vi "Configure Numeric Preset.vi"(8 "error in (no error)":errorcluster, 9 "Preset (Pattern 1)":i32(ring)=1 items=["Pattern 1"=1, "Pattern 2"=2, "Pattern 3"=3, "Pattern 4"=4], 10 "Target Item (0: Normal)":i32(ring) items=["Normal", "Harmonics"], 11 "VISA resource name":refnum<visa-resource-name>) -> (0 "error out":errorcluster, 3 "VISA resource name out":refnum<visa-resource-name>)   [LabVIEW 2021, in "Yokogawa WT1800 Series.lvlib"]
doc: "Configures the numeric preset features."
uses:
  <instrlib>/Yokogawa WT1800 Series/Yokogawa WT1800 Series.lvlib
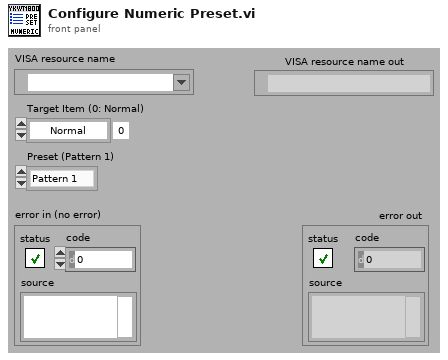
[diagram p1: front panel]
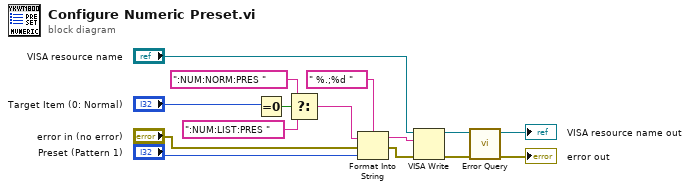
[diagram p0: block diagram]
diagram:
  n1 = Equal To 0?(x="Target Item (0: Normal)") -> (x = 0?=w3:bool)
  n2 = Select(t=":NUM:NORM:PRES " ("形式文字列"), s=w3, f=":NUM:LIST:PRES " ("形式文字列")) -> (s? t:f=w1:string)
  n3 = Format Into String(format string=" %.;%d " ("形式文字列"), initial string=w1, error in="error in (no error)", "Preset (Pattern 1)") -> (resulting string=w6:string, error out=w7:errorcluster)
  n4 = VISA Write ("VISA書き込み")(VISA resource name="VISA resource name", write buffer=w6, error in (no error)=w7) -> (VISA resource name out=w15:refnum<visa-resource-name>, error out=w14:errorcluster)  [unwired: 1 out]
  n5 = call <instrlib>:"Error Query.vi"("error in (no error)"=w14, "VISA resource name"=w15) -> ("error out"=→"error out":errorcluster, "VISA resource name out"=→"VISA resource name out":refnum<visa-resource-name>)  [unwired: 6 in, 2 out]
